vi "ingest.video_new.vi"(8 "error in":errorcluster, 11 "VideoCreateStaging in":refnum<class "VideoCreateStaging.lvclass">) -> (0 "error out":errorcluster, 3 "VideoCreateStaging out":refnum<class "VideoCreateStaging.lvclass">)   [LabVIEW 2020, in "VideoCreateStaging.lvclass"]
doc: "Ingests a standalone video file into a newly created video resource, given its start time."
uses:
  VideoCreateStaging.lvclass
  VideoCreateStaging.lvclass/VideoCreateStaging.ctl
  client.lvlib
panel:
  out "out_job out":i32
  in  "file_path":string
  in  "video_create":i32
  in  "start_ms":dbl
  in  "out_job":i32
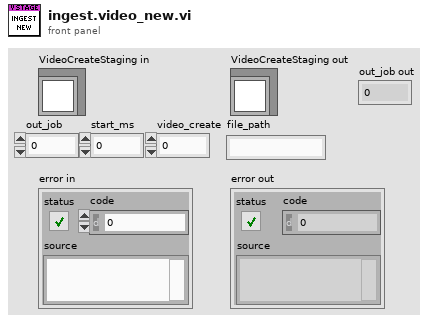
[diagram p1: front panel]
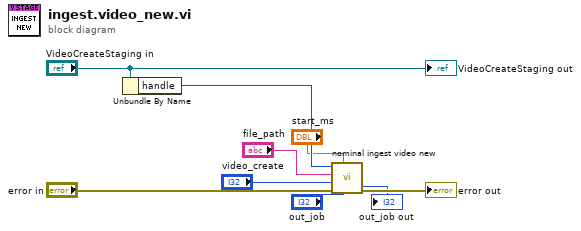
[diagram p0: block diagram]
diagram:
  n1 = Unbundle By Name("VideoCreateStaging in") -> ("handle"=w7:i32)
  n2 = call "nominal ingest video new.vi"("out_job"="out_job", "start_ms"="start_ms", "error in (no error)"="error in", "video_create"="video_create", "file_path"="file_path", "client"=w7) -> ("error out"=→"error out":errorcluster, "out_job out"=→"out_job out":i32)  [unwired: 3 in, 1 out]
  "VideoCreateStaging out" <- "VideoCreateStaging in"
